vi "Close.vi"(8 "error in":errorcluster, 11 "com in":refnum<visa-resource-name>) -> (0 "error out":errorcluster)   [LabVIEW 2020]
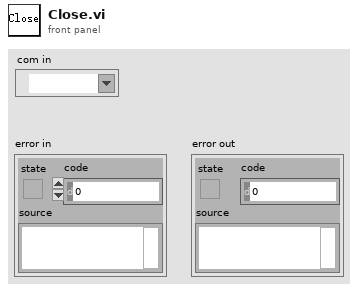
[diagram p1: front panel]
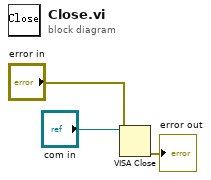
[diagram p0: block diagram]
diagram:
  n1 = VISA Close(VISA resource name="com in", error in (no error)="error in") -> (error out=→"error out":errorcluster)
